vi "Start Sync.vi"(8 "error in (no error)":errorcluster, 11 "gRPC service in":refnum<class "OOBgRPCService.lvclass">) -> (0 "error out":errorcluster, 3 "gRPC service out":refnum<class "OOBgRPCService.lvclass">)   [LabVIEW 2025, in "OOB gRPC Server.lvlib" / "OOBgRPCService.lvclass"]
uses:
  OOBgRPCService.lvclass
  OOBgRPCService.lvclass/OOBgRPCService.ctl
  RPC Messages/hwval_GenericResponse.ctl
  CAN-LIN Frame Generator UI/XNET Frame Type CAN.ctl
  RPC Messages/hwval_StatusResponse.ctl
  OOB Data Transfer/OOB Data Transfer.lvlib
  OOB gRPC Server.lvlib
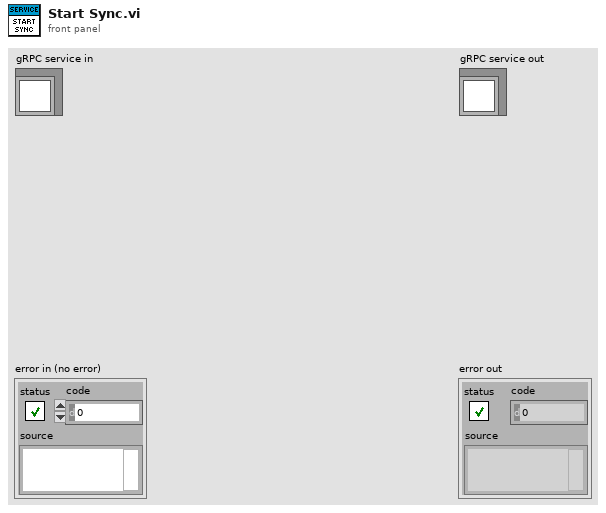
[diagram p1: front panel]
types:
  T1 = typedef "OOB gRPC Server.lvlib/hwval_GenericResponse.ctl" = cluster{"Payload":u8[]}
  T2 = typedef "OOB gRPC Server.lvlib/hwval_StatusResponse.ctl" = cluster{"Status":bool, "Code":i32, "Message":string}
  T3 = typedef "OOB gRPC Server.lvlib/OOBgRPCService.lvclass/Server Internal UEs.ctl" = cluster{"OOBgRPCService Generic Internal UE":refnum<user-event>, "OOBgRPCService PauseResume Internal UE":refnum<user-event>, "OOBgRPCService Export Internal UE":refnum<user-event>}
  T4 = typedef "OOB gRPC Server.lvlib/OOBgRPCService.lvclass/Server gRPC UEs.ctl" = cluster{"OOBgRPCService Generic gRPC UE":refnum<user-event>, "OOBgRPCService PauseResume gRPC UE":refnum<user-event>, "OOBgRPCService Export gRPC UE":refnum<user-event>}
  T5 = typedef "grpc-lvsupport-release.lvlib/grpcId.ctl" = u64
  T6 = typedef "OOB gRPC Server.lvlib/hwval_GenericRequest.ctl" = cluster{"Command":string, "Payload":u8[]}
  T7 = typedef "OOB Data Transfer.lvlib/OOB to Logic Data.ctl" = cluster{"PauseResume":bool, "Export":string, "IDENTIFIER":u32, "TYPE":T8, "DLC":u32, "SEND":bool, "PAYLOAD":u32[], "IDENTIFIER 2":u32, "DLC 2":u32, "SEND 2":bool, "PAYLOAD 2":u32[], "out_str":string}
  T8 = typedef "XNET Frame Type CAN.ctl" = u32
  T9 = typedef "OOB gRPC Server.lvlib/hwval_BoolRequest.ctl" = cluster{"BooleanData":bool}
  T10 = typedef "OOB gRPC Server.lvlib/hwval_ExportRequest.ctl" = cluster{"FileType":string}
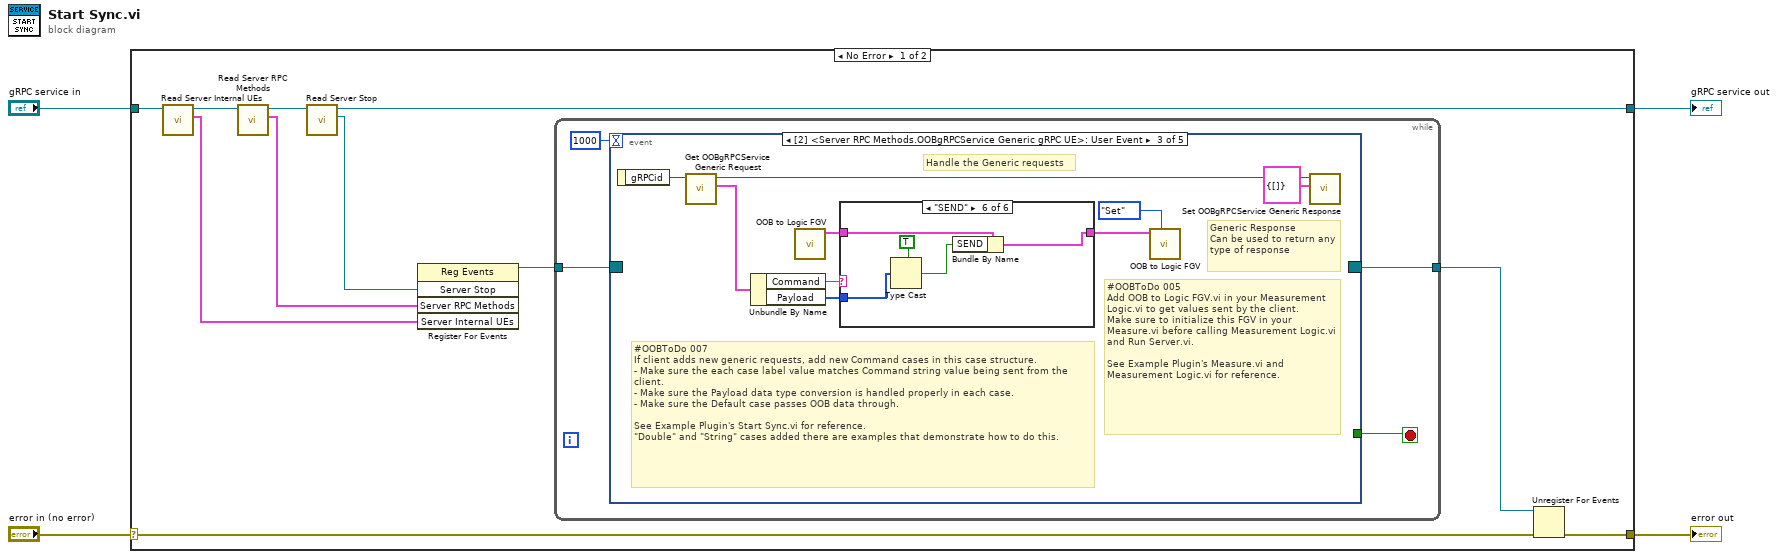
[diagram p0: block diagram]
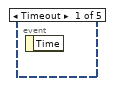
[diagram p2: hidden frame]
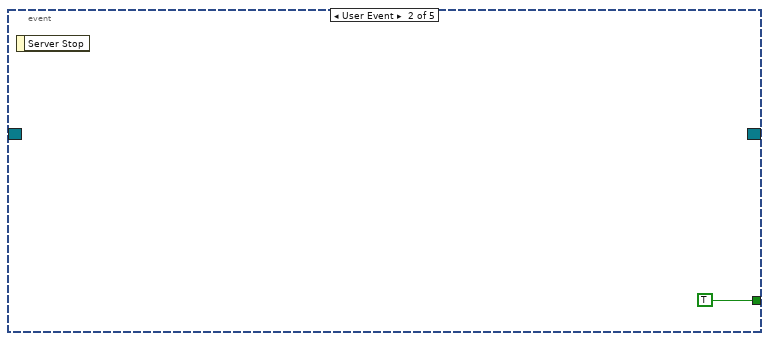
[diagram p3: hidden frame]
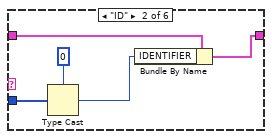
[diagram p5: hidden frame]
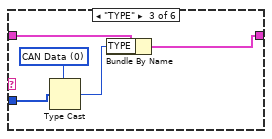
[diagram p6: hidden frame]
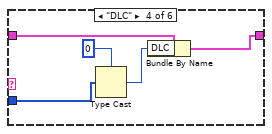
[diagram p7: hidden frame]
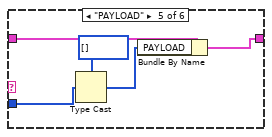
[diagram p8: hidden frame]
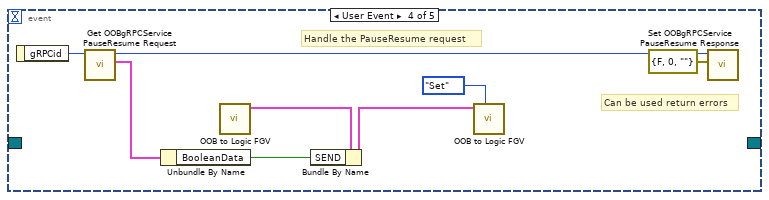
[diagram p9: hidden frame]
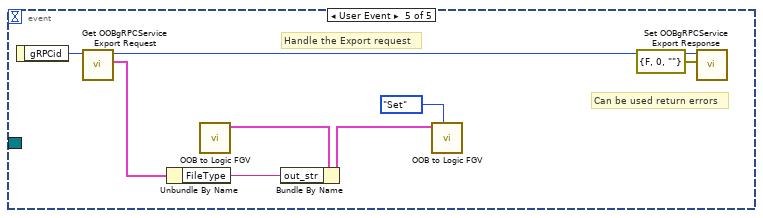
[diagram p10: hidden frame]
diagram:
  n1 = case shown="No Error" "error in (no error)" {
    selector: "error in (no error)" -> [w9 w73]
    tunnel: [w8 w73] -> w3
    tunnel: [w6 w72] -> w1
    tunnel: "gRPC service in" -> [w15 w72]
    frame No Error {
      n2 = call "Read Server Internal UEs.vi"("gRPC service in"=w15) -> ("Server Internal UEs"=w13:T3, "gRPC service out"=w14:refnum<class "OOBgRPCService.lvclass">)  [unwired: 8 in, 1 out]
      n3 = call "Read Server RPC Methods.vi"("gRPC service in"=w14) -> ("Server RPC Methods"=w7:T4, "gRPC service out"=w12:refnum<class "OOBgRPCService.lvclass">)  [unwired: 8 in, 1 out]
      n4 = call-dynamic "Read Server Stop.vi"("gRPC service in"=w12) -> ("Server Stop"=w5:refnum<user-event>, "gRPC service out"=w6:refnum<class "OOBgRPCService.lvclass">)  [unwired: 8 in, 1 out]
      n5 = register-events(w5, w7, w13) -> (reference out=w11:refnum<event-registration>)  [unwired: 2 in, 1 out]
      n6 = while {
        tunnel: w11 -> [w19]
        tunnel: [w17] -> w10
        stop <- w18 stop-if-true
        n7 = event "RPC Methods Event Structure" shown="[2] <Server RPC Methods.OOBgRPCService Generic gRPC UE>: User Event" {
          selector: w19 -> [_ _ _ _ _]
          dyn-events: [_ _ _ _ _] -> w17
          timeout: 1000 -> [_ _ _ _ _]
          tunnel: [_ TRUE _ _ _] -> w18
          event Timeout {
            n8 = event-data() -> ()  [unwired: 1 in, 1 out]
          }
          event User Event {
            n9 = event-data() -> ()  [unwired: 1 in, 1 out]
          }
          event User Event {
            # "#OOBToDo 007 \nIf client adds new generic requests, add new Command cases in this case structure. \n- Make sure the each case label value matches Command string value being sent from the client.\n- Make sure the Payload data type conversion is handled properly in each case.\n- Make sure the Default case passes OOB data through.\n\nSee Example Plugin's Start Sync.vi for reference. \n\"Double\" and \"String\" cases added there are examples that demonstrate how to do this."
            # "Handle the Generic requests"
            # "Generic Response\nCan be used to return any type of response"
            # "#OOBToDo 005 \nAdd OOB to Logic FGV.vi in your Measurement Logic.vi to get values sent by the client.\nMake sure to initialize this FGV in your Measure.vi before calling Measurement Logic.vi and Run Server.vi.\n\nSee Example Plugin's Measure.vi and Measurement Logic.vi for reference."
            n10 = event-data() -> ("gRPCid"=w29:T5)  [unwired: 1 in]
            n11 = call "Get OOBgRPCService Generic Request.vi"("gRPCid"=w29) -> ("Message Data"=w27:T6, "gRPCid out"=w28:T5)  [unwired: 8 in, 1 out]
            n12 = Unbundle By Name(w27) -> ("Command"=w22:string, "Payload"=w21:u8[])
            n13 = call "OOB to Logic FGV.vi"() -> ("OOB to Logic Data out"=w24:T7)  [unwired: 10 in, 1 out]
            n14 = case shown="\"SEND\"" w22 {
              tunnel: w24 -> [w30 w35 w40 w45 w50 w55]
              tunnel: [w30 w34 w39 w44 w49 w54] -> w23
              tunnel: w21 -> [_ w33 w36 w41 w47 w51]
              frame Default {
              }
              frame "ID" {
                n15 = Type Cast(type=u32 0 ("IDENTIFIER"), x=w33) -> (*(type *) &x=w31:u32)
                n16 = Bundle By Name(cluster=w35, "IDENTIFIER"=w31) -> (w34:T7)
              }
              frame "TYPE" {
                w38 = T8 0 items=["CAN Data"=0, "CAN Remote"=1, "CAN Bus Error"=2, "CAN 2.0 Data"=8, "CAN FD Data"=16, "CAN FD+BRS Data"=24, "J1939 Data"=192, "Delay"=224, "Log Trigger"=225, "Start Trigger"=226] ("TYPE")
                n17 = Type Cast(type=w38, x=w36) -> (*(type *) &x=w37:T8)
                n18 = Bundle By Name(cluster=w40, "TYPE"=w37) -> (w39:T7)
              }
              frame "DLC" {
                n19 = Type Cast(type=u32 0 ("DLC"), x=w41) -> (*(type *) &x=w42:u32)
                n20 = Bundle By Name(cluster=w45, "DLC"=w42) -> (w44:T7)
              }
              frame "PAYLOAD" {
                n21 = Type Cast(type=u32[] [] ("PAYLOAD"), x=w47) -> (*(type *) &x=w46:u32[])
                n22 = Bundle By Name(cluster=w50, "PAYLOAD"=w46) -> (w49:T7)
              }
              frame "SEND" {
                n23 = Type Cast(type=TRUE, x=w51) -> (*(type *) &x=w52:bool)
                n24 = Bundle By Name(cluster=w55, "SEND"=w52) -> (w54:T7)
              }
            }
            n25 = call "OOB to Logic FGV.vi"("Op (Get)"=enum16{"Get", "Set"}."Set", "OOB to Logic Data in"=w23) -> ()  [unwired: 8 in, 2 out]
            n26 = call "Set OOBgRPCService Generic Response.vi"("Message Data"=T1 {"Payload"=[]}, "gRPCid in"=w28) -> ()  [unwired: 9 in, 1 out]
          }
          event User Event {
            # "Handle the PauseResume request"
            # "Can be used return errors"
            n27 = event-data() -> ("gRPCid"=w57:T5)  [unwired: 1 in]
            n28 = call "Get OOBgRPCService PauseResume Request.vi"("gRPCid"=w57) -> ("Message Data"=w59:T9, "gRPCid out"=w60:T5)  [unwired: 8 in, 1 out]
            n29 = Unbundle By Name(w59) -> ("BooleanData"=w58:bool)
            n30 = call "OOB to Logic FGV.vi"() -> ("OOB to Logic Data out"=w62:T7)  [unwired: 10 in, 1 out]
            n31 = Bundle By Name(cluster=w62, "SEND"=w58) -> (w61:T7)
            n32 = call "OOB to Logic FGV.vi"("Op (Get)"=enum16{"Get", "Set"}."Set", "OOB to Logic Data in"=w61) -> ()  [unwired: 8 in, 2 out]
            n33 = call "Set OOBgRPCService PauseResume Response.vi"("Message Data"=T2 {"Status"=FALSE, "Code"=0, "Message"=""}, "gRPCid in"=w60) -> ()  [unwired: 9 in, 1 out]
          }
          event User Event {
            # "Handle the Export request"
            # "Can be used return errors"
            n34 = event-data() -> ("gRPCid"=w65:T5)  [unwired: 1 in]
            n35 = call "Get OOBgRPCService Export Request.vi"("gRPCid"=w65) -> ("Message Data"=w67:T10, "gRPCid out"=w71:T5)  [unwired: 8 in, 1 out]
            n36 = Unbundle By Name(w67) -> ("FileType"=w66:string)
            n37 = call "OOB to Logic FGV.vi"() -> ("OOB to Logic Data out"=w69:T7)  [unwired: 10 in, 1 out]
            n38 = Bundle By Name(cluster=w69, "out_str"=w66) -> (w68:T7)
            n39 = call "OOB to Logic FGV.vi"("Op (Get)"=enum16{"Get", "Set"}."Set", "OOB to Logic Data in"=w68) -> ()  [unwired: 8 in, 2 out]
            n40 = call "Set OOBgRPCService Export Response.vi"("Message Data"=T2 {"Status"=FALSE, "Code"=0, "Message"=""}, "gRPCid in"=w71) -> ()  [unwired: 9 in, 1 out]
          }
        }
      }
      n41 = Unregister For Events(event registration refnum=w10, error in=w9) -> (error out=w8:errorcluster)
    }
    frame Error {
    }
  }
  "error out" <- w3
  "gRPC service out" <- w1
